vi "Matlab Param Array to Boolean.vi"(8 "error in (no error)":errorcluster, 10 "Name":string, 11 "Matlab Param Array":cluster{"Name":string, "Data":variant}[](array[cluster])) -> (0 "error out":errorcluster, 3 "data":bool)   [LabVIEW 2014, in "Matlab API.lvlib"]
uses:
  Matlab API.lvlib
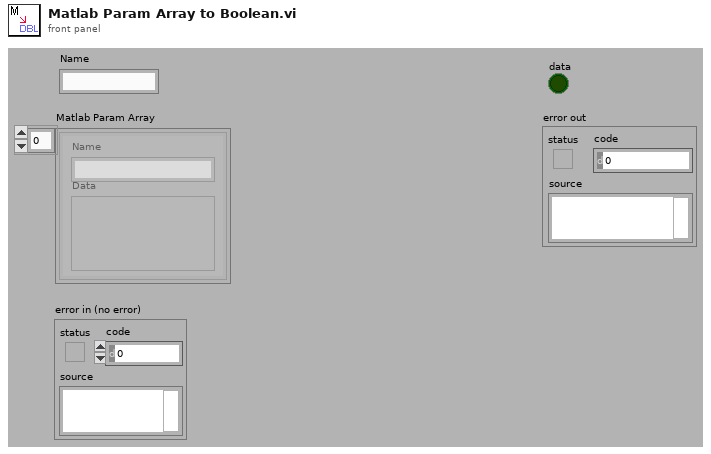
[diagram p1: front panel]
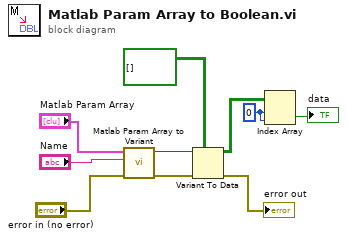
[diagram p0: block diagram]
diagram:
  w3 = 0 ("index (row)")
  n1 = call "Matlab Param Array to Variant.vi"("error in (no error)"="error in (no error)", "Name"="Name", "Variables"="Matlab Param Array") -> ("error out"=w9:errorcluster, "Data"=w10:variant)  [unwired: 7 out]
  n2 = Variant To Data(error in=w9, type=bool[][] [] ("Array"), Variant=w10) -> (data=w4:bool[][], error out=→"error out":errorcluster)
  n3 = Index Array(array=w4, index (row)=w3, index (col)=w3) -> (element=→"data":bool)
